vi "Close DB Reference.vi"(8 "error in (no error)":errorcluster, 11 "Access in":refnum<class "Access.lvclass">) -> (0 "error out":errorcluster, 3 "Access out":refnum<class "Access.lvclass">)   [LabVIEW 2021, in "Database.lvlib" / "Access.lvclass"]
uses:
  Access.lvclass
  Access.lvclass/Access.ctl
  <vilib>/addons/database/Connection.llb/Conn ObjectReference.ctl
  <vilib>/addons/database/NI_Database_API.lvlib
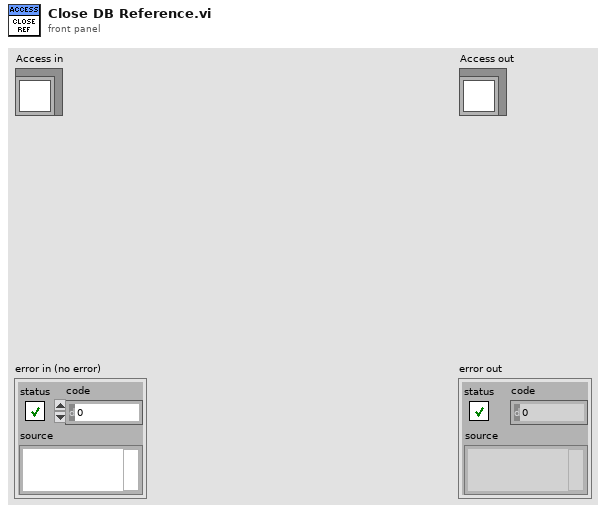
[diagram p1: front panel]
types:
  T1 = typedef "NI_Database_API.lvlib/Conn ObjectReference.ctl" = refnum<k1>
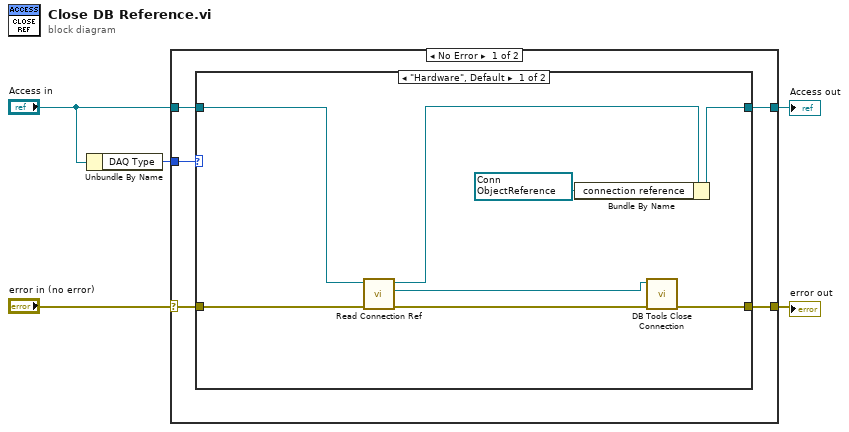
[diagram p0: block diagram]
diagram:
  n1 = Unbundle By Name("Access in") -> ("DAQ Type"=w2:enum16{"Hardware", "Simulation"})
  n2 = case shown="No Error" "error in (no error)" {
    selector: "error in (no error)" -> [w10 w21]
    tunnel: [w9 w22] -> w5
    tunnel: [w8 w21] -> w4
    tunnel: "Access in" -> [w7 w22]
    tunnel: w2 -> [w6 _]
    frame No Error {
      n3 = case shown="\"Hardware\", Default" w6 {
        tunnel: w10 -> [w11 w19]
        tunnel: [w18 w20] -> w9
        tunnel: [w17 w19] -> w8
        tunnel: w7 -> [w16 w20]
        frame "Hardware", Default {
          w13 = T1 refnum items=["Connection"] ("connection reference")
          n4 = call-dynamic "Read Connection Ref.vi"("error in (no error)"=w11, "Access in"=w16) -> ("error out"=w15:errorcluster, "connection reference"=w14:T1, "Access out"=w12:refnum<class "Access.lvclass">)  [unwired: 7 in]
          n5 = Bundle By Name(cluster=w12, "connection reference"=w13) -> (w18:refnum<class "Access.lvclass">)
          n6 = call <vilib>:"DB Tools Close Connection.vi"("error in (no error)"=w15, "connection reference"=w14) -> ("error out"=w17:errorcluster)  [unwired: 5 in]
        }
        frame "Simulation" {
        }
      }
    }
    frame Error {
    }
  }
  "error out" <- w4
  "Access out" <- w5
